vi "Execute.Async.vi"(10 "parameters":variant, 11 "process":refnum<class "Process.lvclass">) -> ()   [LabVIEW 2020, in "Ballard ARINC 429 Engine.lvlib" / "Custom Device.lvlib"]
uses:
  Custom Device.lvlib
  <vilib>/NI/NIVS Inline Async API/_VS Inline Async API/Process/Process.lvclass
  Asynchronous Process Parameters.ctl
  Asynchronous Execution Unit Runtime Information.ctl
  Interfaces/Execution Unit/Execution Unit.lvclass
  Interfaces/Shared Resources/Shared Resources.lvclass
  <vilib>/NI/NIVS Inline Async API/_VS Inline Async API/Process/Process.lvclass/Process.ctl
  <vilib>/NI/NIVS Inline Async API/_Data Access Engine/Access Type Classes/ReadWrite/ReadWrite.lvclass/ReadWrite.ctl
  <vilib>/NI/NIVS Inline Async API/_Data Access Engine/Access Type Classes/Read/Read.lvclass/Read.ctl
  <vilib>/NI/NIVS Inline Async API/_Data Access Engine/Access Type Classes/Write/Write.lvclass/Write.ctl
  <vilib>/NI/NIVS Inline Async API/_Data Access Engine/Data Access Engine/Methods/Read.Data.vi
  <vilib>/NI/NIVS Inline Async API/_Data Access Engine/Data Access Engine/Methods/Write.Data.vi
  <vilib>/NI/NIVS Inline Async API/_Data Access Engine/Data Access Engine/Methods/ReadWrite.Data.vi
  <vilib>/NI/NIVS Inline Async API/_VS Inline Async API/Process/Data Member Access/Read Data Access.vi
  <vilib>/NI/NIVS Inline Async API/_VS Inline Async API/Error Handling Process/SubVIs/Error.ConvertArray.vi
  <vilib>/NI/NIVS Inline Async API/_Data Access Engine/Access Type Classes/Read/Read.ProcessData.vi
  <vilib>/NI/NIVS Inline Async API/_Data Access Engine/Access Type Classes/Write/Write.ProcessData.vi
  <vilib>/NI/NIVS Inline Async API/_Data Access Engine/Access Type Classes/ReadWrite/ReadWrite.ProcessData.vi
  <vilib>/NI/NIVS Inline Async API/_Data Access Engine/Access Type Classes/Write/Write.Buffer.vi
  <vilib>/NI/NIVS Inline Async API/_Data Access Engine/Access Type Classes/Write/Write.Commit.vi
  <vilib>/NI/NIVS Inline Async API/_Data Access Engine/Data Access Engine/Methods/Write.Lookup.vi
  <vilib>/NI/NIVS Inline Async API/_Data Access Engine/Data Access Engine/Methods/ReadWrite.Lookup.vi
  <vilib>/NI/NIVS Inline Async API/_Data Access Engine/Data Access Engine/Methods/Read.Lookup.vi
  <vilib>/NI/NIVS Inline Async API/_Data Access Engine/Data Access Engine/Data Access Engine.lvclass
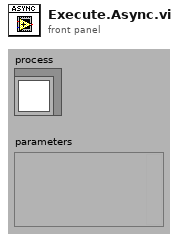
[diagram p1: front panel]
types:
  T1 = typedef "Asynchronous Process Parameters.ctl" = cluster{"Asynchronous Execution Unit Runtime Information":T2, "shared resources":refnum<class "Shared Resources.lvclass">}
  T2 = typedef "Ballard ARINC 429 Engine.lvlib/Custom Device.lvlib/Asynchronous Execution Unit Runtime Information.ctl" = cluster{"Execution Unit":refnum<class "Execution Unit.lvclass">, "Incoming Channel Group Name":string, "Outgoing Channel Group Name":string, "ReadWrite Channel Group Name":string}
  T3 = typedef "Data Access Engine.lvlib/Data Access Engine.lvclass/Write.DVR.ctl" = refnum<data-value>
  T4 = typedef "Data Access Engine.lvlib/Data Access Engine.lvclass/ReadWrite.DVR.ctl" = refnum<data-value>
  T5 = typedef "Data Access Engine.lvlib/Data Access Engine.lvclass/Read.DVR.ctl" = refnum<data-value>
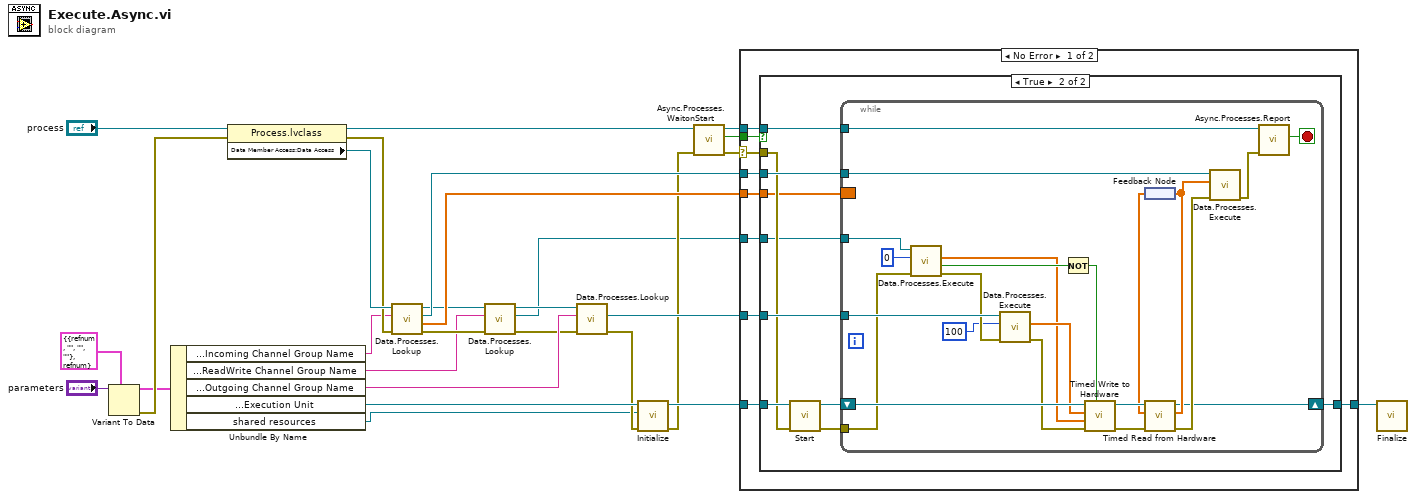
[diagram p0: block diagram]
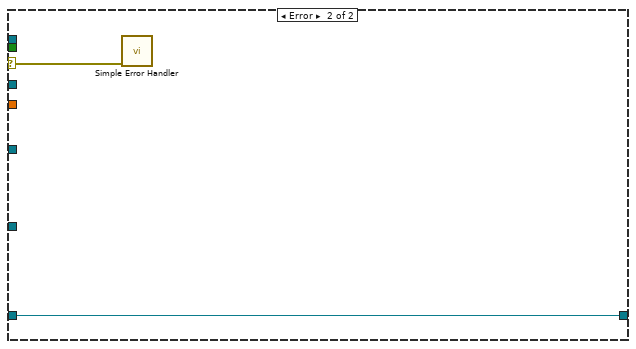
[diagram p3: hidden frame]
diagram:
  n1 = Variant To Data(type=T1 {"Asynchronous Execution Unit Runtime Information"={"Execution Unit"=refnum, "Incoming Channel Group Name"="", "Outgoing Channel Group Name"="", "ReadWrite Channel Group Name"=""}, "shared resources"=refnum} ("asynchronous process parameters"), Variant="parameters") -> (data=w17:T1, error out=w18:errorcluster)  [unwired: 1 in]
  n2 = Unbundle By Name(w17) -> ("Asynchronous Execution Unit Runtime Information.Incoming Channel Group Name"=w16:string, "Asynchronous Execution Unit Runtime Information.ReadWrite Channel Group Name"=w1:string, "Asynchronous Execution Unit Runtime Information.Outgoing Channel Group Name"=w15:string, "Asynchronous Execution Unit Runtime Information.Execution Unit"=w13:refnum<class "Execution Unit.lvclass">, "shared resources"=w7:refnum<class "Shared Resources.lvclass">)
  n3 = property class="Process.lvclass"(reference="process", error in=w18) -> (reference out=w22:refnum<class "Process.lvclass">, error out=w20:errorcluster, "Data Member Access:Data Access"=w21:refnum<class "Data Access Engine.lvclass">)
  n4 = call-poly <vilib>:"Data.Processes.Lookup.vi"("error in (no error)"=w20, "Name"=w16, "Data Access API in"=w21) -> ("error out"=w6:errorcluster, "Initial Values"=w14:dbl[], "Ref"=w24:T3, "Data Access API out"=w5:refnum<class "Data Access Engine.lvclass">)  [unwired: 5 in]
  n5 = call-poly <vilib>:"Data.Processes.Lookup.vi"("error in (no error)"=w6, "Name"=w1, "Data Access API in"=w5) -> ("error out"=w3:errorcluster, "Ref"=w2:T4, "Data Access API out"=w4:refnum<class "Data Access Engine.lvclass">)  [unwired: 5 in, 1 out]
  n6 = call-poly <vilib>:"Data.Processes.Lookup.vi"("error in (no error)"=w3, "Name"=w15, "Data Access API in"=w4) -> ("error out"=w11:errorcluster, "Ref"=w25:T5)  [unwired: 5 in, 2 out]
  n7 = call-dynamic "Initialize.vi"("error in"=w11, "shared resources"=w7, "Execution Unit in"=w13) -> ("error out"=w10:errorcluster, "Execution Unit out"=w12:refnum<class "Execution Unit.lvclass">)  [unwired: 7 in]
  n8 = call <vilib>:"Async.Processes.WaitonStart.vi"("error in (no error)"=w10, "Process"=w22) -> ("error out"=w26:errorcluster, "Execute"=w28:bool, "Process out"=w27:refnum<class "Process.lvclass">)  [unwired: 7 in]
  n9 = case shown="No Error" w26 {
    selector: w26 -> [w33 w72]
    tunnel: w28 -> [w37 _]
    tunnel: w27 -> [w36 _]
    tunnel: w24 -> [w35 _]
    tunnel: w25 -> [w34 _]
    tunnel: w14 -> [w32 _]
    tunnel: w12 -> [w31 w71]
    tunnel: [w30 w71] -> w9
    tunnel: w2 -> [w29 _]
    frame No Error {
      n10 = case shown="True" w37 {
        tunnel: w33 -> [_ w44]
        tunnel: w36 -> [_ w46]
        tunnel: w34 -> [_ w48]
        tunnel: w35 -> [_ w47]
        tunnel: w32 -> [_ w41]
        tunnel: w31 -> [w38 w45]
        tunnel: [w38 w40] -> w30
        tunnel: w29 -> [_ w39]
        frame False {
        }
        frame True {
          n11 = call-dynamic "Start.vi"("error in (no error)"=w44, "Execution Unit in"=w45) -> ("error out"=w43:errorcluster, "Execution Unit out"=w42:refnum<class "Execution Unit.lvclass">)  [unwired: 8 in]
          n12 = while {
            tunnel: w43 -> [w57]
            tunnel: w46 -> [w70]
            tunnel: w48 -> [w68]
            tunnel: w47 -> [w67]
            border: w41 -> [_]
            shift-right: [w60] -> w40
            shift-left: w42 -> [w66]
            tunnel: w39 -> [w59]
            stop <- w69 stop-if-true
            n13 = call-poly <vilib>:"Data.Processes.Execute.vi"("error in (no error)"=w57, "timeout ms"=0, "Ref"=w59) -> ("error out"=w56:errorcluster, "Timeout?"=w53:bool, "Data"=w49:dbl[])  [unwired: 5 in, 1 out]
            n14 = call-poly <vilib>:"Data.Processes.Execute.vi"("error in (no error)"=w56, "timeout ms"=100, "Ref"=w68) -> ("error out"=w64:errorcluster, "Values"=w50:dbl[])  [unwired: 6 in, 1 out]
            n15 = Not(x=w53) -> (.not. x?=w51:bool)
            n16 = call "Timed Write to Hardware.vi"("Valid triggers"=w51, "error in"=w64, "Trigger Values"=w49, "Values"=w50, "Execution Unit in"=w66) -> ("error out"=w54:errorcluster, "Execution Unit out"=w65:refnum<class "Execution Unit.lvclass">)  [unwired: 3 in, 2 out]
            n17 = feedback #1() -> (w62:dbl[])
            n18 = call "Timed Read from Hardware.vi"("error in"=w54, "Values in"=w62, "Execution Unit in"=w65) -> ("error out"=w63:errorcluster, "Values out"=w61:dbl[], "Execution Unit out"=w60:refnum<class "Execution Unit.lvclass">)  [unwired: 6 in]
            n19 = feedback-in #1(w61) -> ()
            n20 = call-poly <vilib>:"Data.Processes.Execute.vi"("error in (no error)"=w63, "Values"=w61, "Ref"=w67) -> ("error out"=w58:errorcluster)  [unwired: 8 in]
            n21 = call <vilib>:"Async.Processes.Report.vi"("Error"=w58, "Process in"=w70) -> ("Stop"=w69:bool)  [unwired: 8 in, 1 out]
          }
        }
      }
    }
    frame Error {
      n22 = call <vilib>:"Simple Error Handler.vi"("error in (no error)"=w72) -> ()  [unwired: 4 in, 5 out]
    }
  }
  n23 = call-dynamic "Finalize.vi"("Execution Unit in"=w9) -> ()  [unwired: 9 in, 2 out]
